vi "Evaluate Fitness.vi"(8 "error in":errorcluster, 10 "Target Sentence in":refnum<class "IChromosome.lvclass">, 11 "Sentence in":refnum<class "Sentence.lvclass">) -> (0 "error out":errorcluster, 3 "Sentence out":refnum<class "Sentence.lvclass">)   [LabVIEW 2016, in "Sentence.lvclass"]
uses:
  Sentence.lvclass
  C:/Users/J51654/My Projects/Evolutionary Programming/GA Framework/IChromosome/IChromosome.lvclass
  IChromosome/IChromosome.lvclass
  Gene/Character.lvclass
  IChromosome/IChromosome.lvclass/IChromosome.ctl
  Gene/Character.lvclass/Character.ctl
  IGene/IGene.lvclass
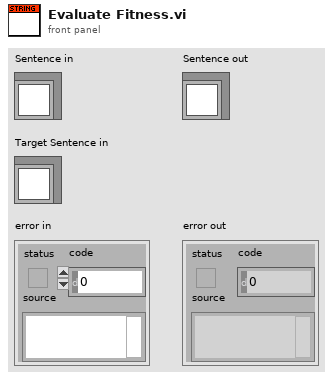
[diagram p1: front panel]
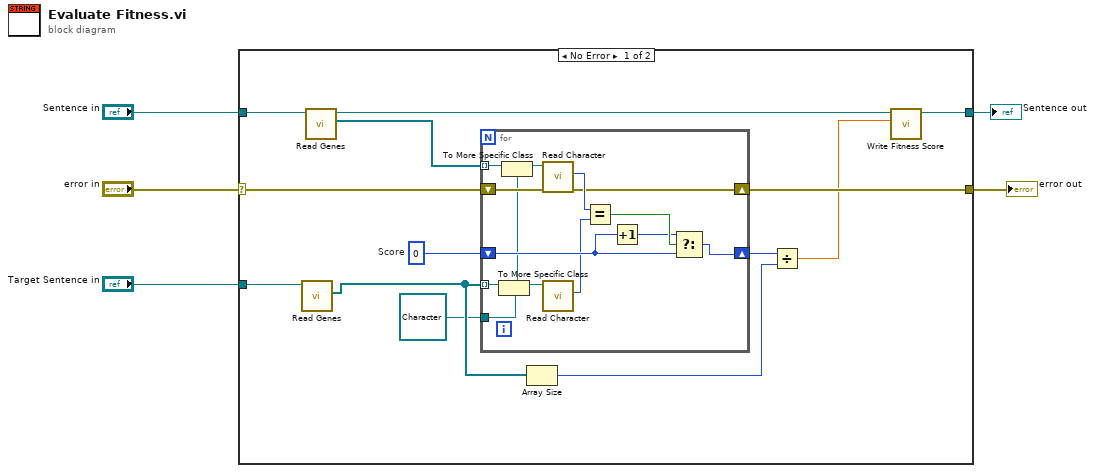
[diagram p0: block diagram]
diagram:
  n1 = case shown="No Error" "error in" {
    selector: "error in" -> [w12 w33]
    tunnel: [w15 w33] -> w5
    tunnel: [w7 w32] -> w4
    tunnel: "Sentence in" -> [w14 w32]
    tunnel: "Target Sentence in" -> [w11 _]
    frame No Error {
      w18 = 0  # Score
      n2 = call "Read Genes.vi"("IChromosome in"=w11) -> ("Genes"=w10:refnum<class "IGene.lvclass">[])  [unwired: 8 in, 2 out]
      n3 = call "Read Genes.vi"("IChromosome in"=w14) -> ("Genes"=w13:refnum<class "IGene.lvclass">[], "IChromosome out"=w8:refnum<class "Sentence.lvclass">)  [unwired: 8 in, 1 out]
      n4 = for {
        tunnel: w13 -> [w23] mode=indexing
        shift-right: [w29] -> w15
        shift-left: w12 -> [w30]
        shift-right: [w25] -> w17
        shift-left: w18 -> [w27]
        tunnel: w10 -> [w21] mode=indexing
        tunnel: refnum<class "Character.lvclass"> refnum ("Character.lvclass") -> [w19]
        n5 = To More Specific Class(target class=w19, reference=w21) -> (specific class reference=w20:refnum<class "Character.lvclass">)  [unwired: 1 in, 1 out]
        n6 = To More Specific Class(target class=w19, reference=w23) -> (specific class reference=w22:refnum<class "Character.lvclass">)  [unwired: 1 in, 1 out]
        n7 = call "Read Character.vi"("error in (no error)"=w30, "Character in"=w22) -> ("error out"=w29:errorcluster, "Character"=w31:u8)  [unwired: 7 in, 1 out]
        n8 = call "Read Character.vi"("Character in"=w20) -> ("Character"=w24:u8)  [unwired: 8 in, 2 out]
        n9 = Equal?(x=w31, y=w24) -> (x = y?=w28:bool)
        n10 = Increment(x=w27) -> (x+1=w26:i32)
        n11 = Select(t=w26, s=w28, f=w27) -> (s? t:f=w25:i32)
      }
      n12 = Array Size(array=w10) -> (size(s)=w16:i32)
      n13 = Divide(x=w17, y=w16) -> (x/y=w6:dbl)
      n14 = call "Write Fitness Score.vi"("Fitness Score"=w6, "IChromosome in"=w8) -> ("IChromosome out"=w7:refnum<class "Sentence.lvclass">)  [unwired: 8 in, 1 out]
    }
    frame Error {
    }
  }
  "error out" <- w5
  "Sentence out" <- w4
